vi "Anritsu VNA Convert INT 16 Data Form 2.vi"(6 "Display Format":T1, 8 "Raw Data Point":string) -> (0 "Number":cdb)   [LabVIEW 2011]
uses:
  tests/S Parameter/TypeDefs/SP Measurement Format.ctl
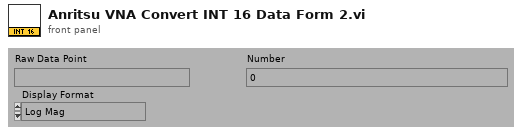
[diagram p1: front panel]
types:
  T1 = typedef "SP Measurement Format.ctl" = enum32{"Log Mag", "Phase", "Delay", "Smith (R+jX)", "Polar (Re/Im)", "Linear Mag", "SWR", "Real", "Imaginary", "Smith (Lin/Phase)", "Smith (Log/Phase)", "Smith (Real/Imag)", "Smith (G+jB)", "Polar (Lin/Phase)", "Polar (Log/Phase)", "Expanded Phase", "Positive Phase", "Inverted Smith", "Unwrapped Phase", "Power Out", "Power In", "Linear Mag/Phase", "Log Mag/Phase", "Real/Imaginary"}
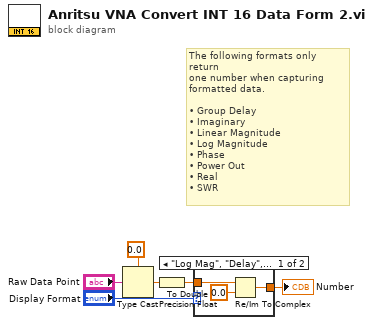
[diagram p0: block diagram]
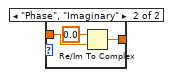
[diagram p2: hidden frame]
diagram:
  # "The following formats only return\none number when capturing\nformatted data.\n\n• Group Delay\n• Imaginary\n• Linear Magnitude\n• Log Magnitude\n• Phase\n• Power Out\n• Real\n• SWR"
  n1 = Type Cast(type=sgl 0.0, x="Raw Data Point") -> (*(type *) &x=w2:sgl)
  n2 = To Double Precision Float(number=w2) -> (double precision float=w4:dbl)
  n3 = case shown="\"Log Mag\", \"Delay\", \"Linear Mag\"..\"Real\", \"Power Out\", Default" "Display Format" {
    tunnel: [w9 w12] -> w5
    tunnel: w4 -> [w8 w11]
    frame "Log Mag", "Delay", "Linear Mag".."Real", "Power Out", Default {
      n4 = Re/Im To Complex(1:0.0 ("y"), 2:w8) -> (0:w9:cdb)
    }
    frame "Phase", "Imaginary" {
      n5 = Re/Im To Complex(1:w11, 2:0.0 ("x")) -> (0:w12:cdb)
    }
  }
  "Number" <- w5
